vi "Untitled 1.vi"() -> ()   [LabVIEW 2023]
uses:
  Classes/Processes/Subclasses/Process Handler/Process Handler.lvclass
panel:
  in  "Checkbox":bool
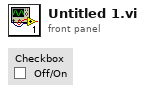
[diagram p1: front panel]
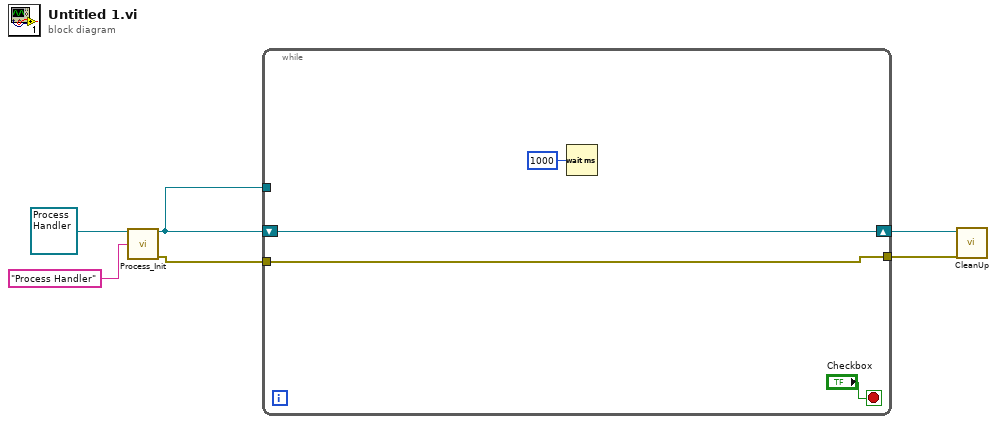
[diagram p0: block diagram]
diagram:
  n1 = call-dynamic "Process_Init.vi"("Process In"=refnum<class "Process Handler.lvclass"> refnum ("Process"), "Process Name"="Process Handler") -> ("Process Out"=w5:refnum<class "Process Handler.lvclass">, "Error Out"=w6:errorcluster)  [unwired: 12 in]
  n2 = while {
    tunnel: w5 -> [_]
    shift-right: [w8] -> w3
    shift-left: w5 -> [w8]
    tunnel: [w9] -> w2
    tunnel: w6 -> [w9]
    stop <- "Checkbox" stop-if-true
    n3 = Wait (ms)(milliseconds to wait=u32 1000) -> ()  [unwired: 1 out]
  }
  n4 = call-dynamic "CleanUp.vi"("Process In"=w3, "Error In"=w2) -> ()  [unwired: 12 in, 2 out]
